vi "Apply (Mono 16 EDVR Buffer).vi"(6 "Mono 16 Buffer Image Size":T1, 7 "Scaling Factor (Default 1.0/256.0)":dbl=0.00390625, 8 "error in (no error)":errorcluster, 9 "Destination Image in":T2, 10 "Mono 16 Buffer in":refnum<data-value>, 11 "CLAHE in":refnum<class "CLAHE.lvclass">) -> (0 "error out":errorcluster, 2 "Destination Image":T2, 3 "CLAHE":refnum<class "CLAHE.lvclass">)   [LabVIEW 2020, in "image.lvlib" / "CLAHE.lvclass"]
uses:
  CLAHE.lvclass
  Greyscale Image.ctl
  common/Image Size (Integer).ctl
  CLAHE.lvclass/CLAHE.ctl
  common/common.lvlib
  common/bin/gartoolkit_32-1.dll
  image.lvlib
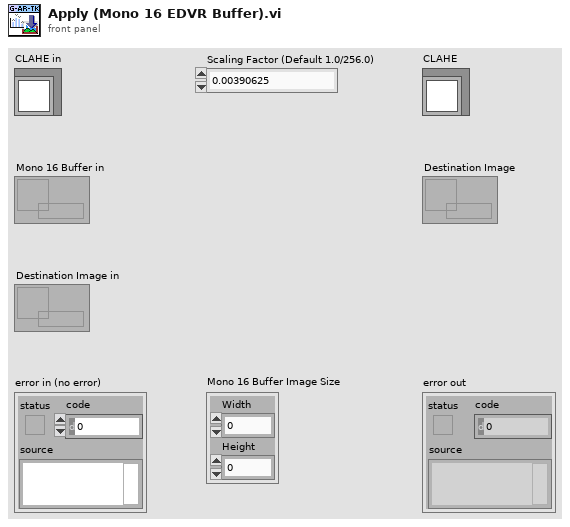
[diagram p1: front panel]
types:
  T1 = typedef "common.lvlib/Image Size (Integer).ctl" = cluster{"Width":u16, "Height":u16}
  T2 = typedef "image.lvlib/Greyscale Image.ctl" = refnum<data-value>
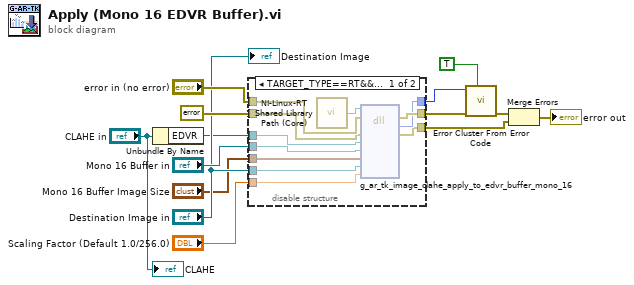
[diagram p0: block diagram]
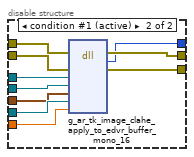
[diagram p2: hidden frame]
diagram:
  n1 = Unbundle By Name("CLAHE in") -> ("EDVR"=w3:refnum<data-value>)
  n2 = disable-structure shown="TARGET_TYPE==RT&&OS==Linux" {
    disable-tunnel: "error in (no error)" -> [w25 w35]
    disable-tunnel: errorcluster {"status"=FALSE, "code"=0, "source"=""} ("error constant") -> [w24 w34]
    disable-tunnel: w3 -> [w23 w30]
    disable-tunnel: [w18 w33] -> w12
    disable-tunnel: [w17 w32] -> w11
    disable-tunnel: [w16 w31] -> w10
    disable-tunnel: "Mono 16 Buffer in" -> [w22 w29]
    disable-tunnel: "Destination Image in" -> [w21 w28]
    disable-tunnel: "Mono 16 Buffer Image Size" -> [w20 w27]
    disable-tunnel: "Scaling Factor (Default 1.0/256.0)" -> [w19 w26]
    frame condition #0 {
      n3 = call "NI-Linux-RT Shared Library Path (Core).vi"() -> ("Path"=w15:path)
      n4 = dll-call lib="?" fn="g_ar_tk_image_clahe_apply_to_edvr_buffer_mono_16" ("g_ar_toolkit.*.*:g_ar_tk_image_copy")(path in=w15, error in=w25, "error_cluster"=w24, "EDVR"=w23, "Source"=w22, "Source Size"=w20, "Destination"=w21, "Scaling Factor"=w19) -> (error out=w18:errorcluster, "return type"=w17:i32, "error_cluster"=w16:errorcluster)  [unwired: 6 in, 1 out]
    }
    frame condition #1 (active) {
      n5 = dll-call lib="C:/serenial/lib/g-augmented-reality-toolkit/LabVIEW/common/bin/gartoolkit_*-1.*" fn="g_ar_tk_image_clahe_apply_to_edvr_buffer_mono_16" ("g_ar_toolkit.*.*:g_ar_tk_image_copy")(error in=w35, "error_cluster"=w34, "EDVR"=w30, "Source"=w29, "Source Size"=w27, "Destination"=w28, "Scaling Factor"=w26) -> (error out=w33:errorcluster, "return type"=w32:i32, "error_cluster"=w31:errorcluster)  [unwired: 7 in, 1 out]
    }
  }
  n6 = call <vilib>:"Error Cluster From Error Code.vi"("show call chain? (False)"=TRUE, "error in (no error)"=w12, "error code (0)"=w11) -> ("error out"=w14:errorcluster)  [unwired: 6 in]
  n7 = Merge Errors(w14, w10) -> (→"error out":errorcluster)
  "CLAHE" <- "CLAHE in"
  "Destination Image" <- "Destination Image in"
